vi "example_01_authorization.vi"() -> ()   [LabVIEW 2015, in "lv-dropbox-examples.lvlib"]
uses:
  lv-dropbox-examples.lvlib
  lv-dropbox/public/_controls/code_challenge_method.ctl
  <vilib>/Utility/error.llb/Error Cluster From Error Code.vi
  <vilib>/Platform/browser.llb/Open URL in Default Browser (string).vi
  <vilib>/ErrorRing/Error Ring.xnode
  lv-dropbox/lv-dropbox.lvlib
panel:
  in  "redirect_uri":string
  in  "code_challenege_method":T1=enum."sha256"
  out "authorization_url":string
  in  "launch_browser":bool
  in  "authorization_code":string
  out "code_verifier":string
  out "error":errorcluster
  out "access_token":string
  in  "app_secret":string
  in  "app_key":string
  in  "access_token":string
  in  "authorization_selection":T2(radio)
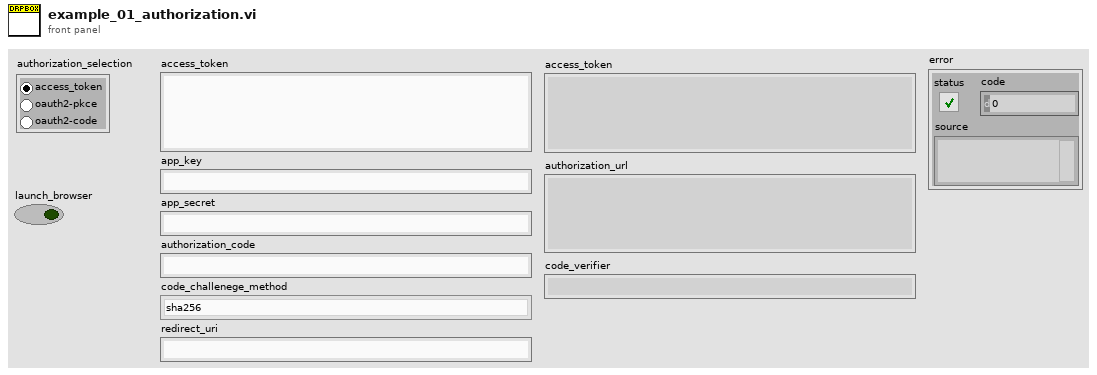
[diagram p1: front panel]
types:
  T1 = typedef "lv-dropbox.lvlib/code_challenge_method.ctl" = enum16{"<challenge_method>", "plain", "sha256"}
  T2 = enum32{"access_token", "oauth2-pkce", "oauth2-code"}
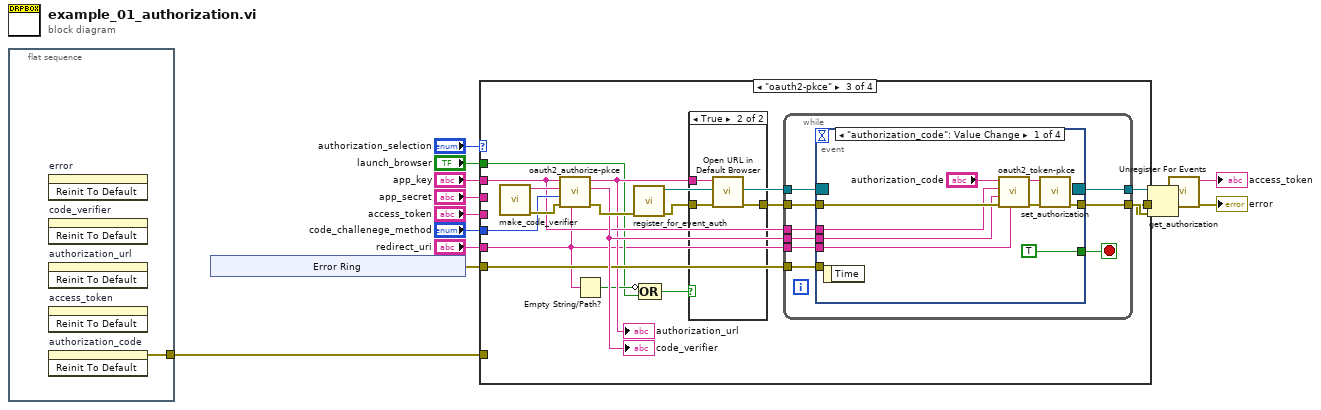
[diagram p0: block diagram]
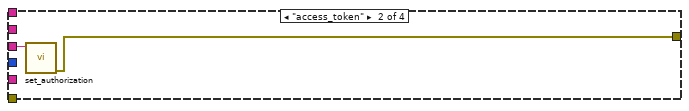
[diagram p3: hidden frame]
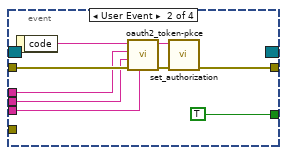
[diagram p5: hidden frame]
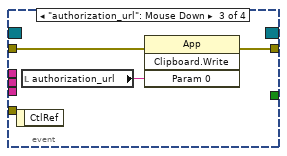
[diagram p6: hidden frame]
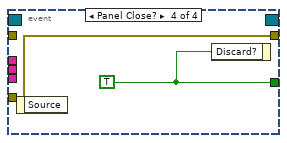
[diagram p7: hidden frame]
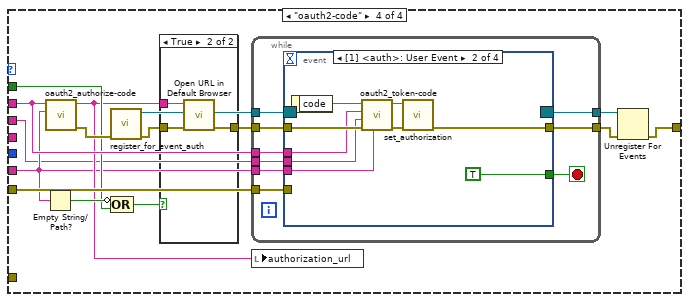
[diagram p8: hidden frame]
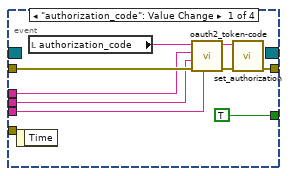
[diagram p10: hidden frame]
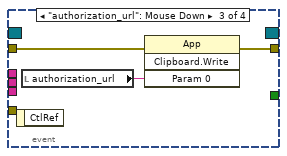
[diagram p11: hidden frame]
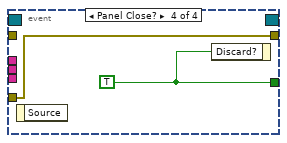
[diagram p12: hidden frame]
diagram:
  n1 = flat-sequence {
    tunnel: [w13] -> w5
    frame #0 {
      n2 = invoke on="error" class="Clust (strict)" method="Reinit To Default"() -> ()  [unwired: 3 in, 3 out]
      n3 = invoke on="code_verifier" class="Str" method="Reinit To Default"() -> ()  [unwired: 3 in, 3 out]
      n4 = invoke on="authorization_url" class="Str" method="Reinit To Default"() -> ()  [unwired: 3 in, 3 out]
      n5 = invoke on="access_token" class="Str" method="Reinit To Default"() -> ()  [unwired: 3 in, 3 out]
      n6 = invoke on="authorization_code" class="Str" method="Reinit To Default"() -> (error out=w13:errorcluster)  [unwired: 3 in, 2 out]
    }
  }
  n7 = xnode "Error Ring"() -> ("error out"=w6:errorcluster)
  n8 = case shown="\"oauth2-pkce\"" "authorization_selection" {
    tunnel: "access_token" -> [_ w15 _ _]
    tunnel: [_ w14 w21 w76] -> w3
    tunnel: "app_key" -> [_ _ w28 w82]
    tunnel: "app_secret" -> [_ _ _ w69]
    tunnel: "launch_browser" -> [_ _ w18 w73]
    tunnel: "code_challenege_method" -> [_ _ w29 _]
    tunnel: w6 -> [_ _ w27 w81]
    tunnel: w5 -> [_ _ _ _]
    tunnel: "redirect_uri" -> [_ _ w16 w70]
    frame Default {
    }
    frame "access_token" {
      n9 = call "set_authorization.vi"("authorization"=w15) -> ("error out"=w14:errorcluster)  [unwired: 10 in]
    }
    frame "oauth2-pkce" {
      n10 = call "make_code_verifier.vi"() -> ("error out"=w31:errorcluster, "code_verifier"=w30:string)  [unwired: 10 in]
      "code_verifier" <- w30
      n11 = call "oauth2_authorize-pkce.vi"("redirect_uri"=w16, "error in (no error)"=w31, "code_challenege_method"=w29, "code_verifier"=w30, "client_id"=w28) -> ("error out"=w32:errorcluster, "auth_url"=w26:string)  [unwired: 5 in]
      "authorization_url" <- w26
      n12 = Empty String/Path?(string/path=w16) -> (empty?=w19:bool)
      n13 = call "register_for_event_auth.vi"("error in (no error)"=w32) -> ("error out"=w24:errorcluster, "event_registration"=w23:refnum<event-registration>)  [unwired: 9 in]
      n14 = Compound Arithmetic op=OR(invert w19, w18) -> (w17:bool)
      n15 = case shown="True" w17 {
        tunnel: w24 -> [w33 w36]
        tunnel: [w33 w35] -> w25
        tunnel: w26 -> [_ w34]
        frame False {
        }
        frame True {
          n16 = call-poly <vilib>:"Open URL in Default Browser.vi"("error in (no error)"=w36, "URL"=w34) -> ("error out"=w35:errorcluster)  [unwired: 4 in, 1 out]
        }
      }
      n17 = while {
        tunnel: w30 -> [w42]
        tunnel: w27 -> [w41]
        tunnel: w28 -> [w43]
        tunnel: w25 -> [w44]
        tunnel: [w45] -> w22
        tunnel: w23 -> [w38]
        tunnel: [w39] -> w20
        tunnel: w16 -> [w37]
        stop <- w40 stop-if-true
        n18 = event shown="[0] \"authorization_code\": Value Change" {
          selector: w38 -> [_ _ _ _]
          dyn-events: [_ _ _ _] -> w39
          timeout: _ -> [_ _ _ _]
          tunnel: [w48 w58 w65 w68] -> w45
          tunnel: w44 -> [w53 w63 w66 _]
          tunnel: w43 -> [w51 w61 _ _]
          tunnel: w42 -> [w52 w62 _ _]
          tunnel: w41 -> [_ _ _ w68]
          tunnel: [TRUE ("done") TRUE ("done") _ w67] -> w40
          tunnel: w37 -> [w46 w55 _ _]
          event "authorization_code": Value Change {
            n19 = event-data() -> ()  [unwired: 1 in, 1 out]
            n20 = call "oauth2_token-pkce.vi"("redirect_uri"=w46, "error in (no error)"=w53, "code_verifier"=w52, "client_id"=w51, "authorization_code"="authorization_code") -> ("error out"=w49:errorcluster, "access_token"=w50:string)  [unwired: 5 in]
            n21 = call "set_authorization.vi"("error in (no error)"=w49, "authorization"=w50) -> ("error out"=w48:errorcluster)  [unwired: 9 in]
          }
          event User Event {
            n22 = event-data() -> ("code"=w56:string)  [unwired: 1 in]
            n23 = call "oauth2_token-pkce.vi"("redirect_uri"=w55, "error in (no error)"=w63, "code_verifier"=w62, "client_id"=w61, "authorization_code"=w56) -> ("error out"=w59:errorcluster, "access_token"=w60:string)  [unwired: 5 in]
            n24 = call "set_authorization.vi"("error in (no error)"=w59, "authorization"=w60) -> ("error out"=w58:errorcluster)  [unwired: 9 in]
          }
          event "authorization_url": Mouse Down {
            n25 = event-data() -> ()  [unwired: 1 in, 1 out]
            n26 = local read "authorization_url"() -> (w64:string)
            n27 = invoke class="App" method="Clipboard.Write"(error in=w66, "Param 0"=w64) -> (error out=w65:errorcluster)  [unwired: 2 in, 3 out]
          }
          event Panel Close? {
            w67 = TRUE ("Discard?")
            n28 = event-data() -> ()  [unwired: 1 in, 1 out]
            n29 = event-data("Discard?"=w67) -> ()  [unwired: 1 in, 1 out]
          }
        }
      }
      n30 = Unregister For Events(event registration refnum=w20, error in=w22) -> (error out=w21:errorcluster)
    }
    frame "oauth2-code" {
      n31 = Empty String/Path?(string/path=w70) -> (empty?=w74:bool)
      n32 = call "oauth2_authorize-code.vi"("redirect_uri"=w70, "client_id"=w82) -> ("error out"=w83:errorcluster, "auth_url"=w71:string)  [unwired: 8 in]
      n33 = call "register_for_event_auth.vi"("error in (no error)"=w83) -> ("error out"=w79:errorcluster, "event_registration"=w78:refnum<event-registration>)  [unwired: 9 in]
      n34 = Compound Arithmetic op=OR(invert w74, w73) -> (w72:bool)
      n35 = case shown="True" w72 {
        tunnel: w79 -> [w84 w87]
        tunnel: [w84 w86] -> w80
        tunnel: w71 -> [_ w85]
        frame False {
        }
        frame True {
          n36 = call-poly <vilib>:"Open URL in Default Browser.vi"("error in (no error)"=w87, "URL"=w85) -> ("error out"=w86:errorcluster)  [unwired: 4 in, 1 out]
        }
      }
      n37 = while {
        tunnel: w70 -> [w93]
        tunnel: w81 -> [w92]
        tunnel: w82 -> [w94]
        tunnel: w80 -> [w95]
        tunnel: [w96] -> w77
        tunnel: w78 -> [w89]
        tunnel: [w90] -> w75
        tunnel: w69 -> [w88]
        stop <- w91 stop-if-true
        n38 = event shown="[1] <auth>: User Event" {
          selector: w89 -> [_ _ _ _]
          dyn-events: [_ _ _ _] -> w90
          timeout: _ -> [_ _ _ _]
          tunnel: [w101 w110 w116 w119] -> w96
          tunnel: w95 -> [w105 w114 w117 _]
          tunnel: w94 -> [w104 w113 _ _]
          tunnel: w93 -> [w98 w107 _ _]
          tunnel: w92 -> [_ _ _ w119]
          tunnel: [TRUE ("done") TRUE ("done") _ w118] -> w91
          tunnel: w88 -> [w97 w106 _ _]
          event "authorization_code": Value Change {
            n39 = event-data() -> ()  [unwired: 1 in, 1 out]
            n40 = local read "authorization_code"() -> (w99:string)
            n41 = call "oauth2_token-code.vi"("redirect_uri"=w98, "error in (no error)"=w105, "client_secret"=w97, "client_id"=w104, "authorization_code"=w99) -> ("error out"=w102:errorcluster, "access_token"=w103:string)  [unwired: 5 in]
            n42 = call "set_authorization.vi"("error in (no error)"=w102, "authorization"=w103) -> ("error out"=w101:errorcluster)  [unwired: 9 in]
          }
          event User Event {
            n43 = event-data() -> ("code"=w108:string)  [unwired: 1 in]
            n44 = call "oauth2_token-code.vi"("redirect_uri"=w107, "error in (no error)"=w114, "client_secret"=w106, "client_id"=w113, "authorization_code"=w108) -> ("error out"=w111:errorcluster, "access_token"=w112:string)  [unwired: 5 in]
            n45 = call "set_authorization.vi"("error in (no error)"=w111, "authorization"=w112) -> ("error out"=w110:errorcluster)  [unwired: 9 in]
          }
          event "authorization_url": Mouse Down {
            n46 = event-data() -> ()  [unwired: 1 in, 1 out]
            n47 = local read "authorization_url"() -> (w115:string)
            n48 = invoke class="App" method="Clipboard.Write"(error in=w117, "Param 0"=w115) -> (error out=w116:errorcluster)  [unwired: 2 in, 3 out]
          }
          event Panel Close? {
            w118 = TRUE ("Discard?")
            n49 = event-data() -> ()  [unwired: 1 in, 1 out]
            n50 = event-data("Discard?"=w118) -> ()  [unwired: 1 in, 1 out]
          }
        }
      }
      n51 = local write "authorization_url"(w71) -> ()
      n52 = Unregister For Events(event registration refnum=w75, error in=w77) -> (error out=w76:errorcluster)
    }
  }
  n53 = call "get_authorization.vi"("error in (no error)"=w3) -> ("error out"=→"error":errorcluster, "authorization"=→"access_token":string)  [unwired: 8 in, 1 out]
